vi "CH_LM App DAQ SendCommand.vi"(4 "error in (no error)":errorcluster, 5 "DAQ Command":T1={"Wait at Rendesvouz"=FALSE, "Command"="", "Sample Collection"=enum."Continuous", "Sample Size"=100, "Collection Mode"=enum."Streaming", "T / ms"=1.0, "NofBins"=7, "Point(s)"=1, "Log Data File"=path "", "Log data to File"=FALSE, "Pause"=FALSE, "Meter Index"=0, "Data format"=0, "Delivery Mode"=enum."Last", "Start/Stop Button"=refnum, "Point(s) Array"=[]} {"Point(s) Array" min=1 max=20000; "Point(s)" min=1 max=20000; "Sample Size" min=1}, 6 "rendezvous":T3, 7 "i ref":refnum<vi>) -> (0 "error out":errorcluster, 2 "timed out":bool, 3 "i ref":refnum<vi>)   [LabVIEW 2012, in "CH_LM App.lvlib"]
doc: "This VI can be used to send a command to the DAQ thread."
uses:
  CH_LM App.lvlib
  CH_LM App DAQ Command.ctl
  CH_LM/CH_LM Measurement Delivery Mode.ctl
  CH_LM.lvlib
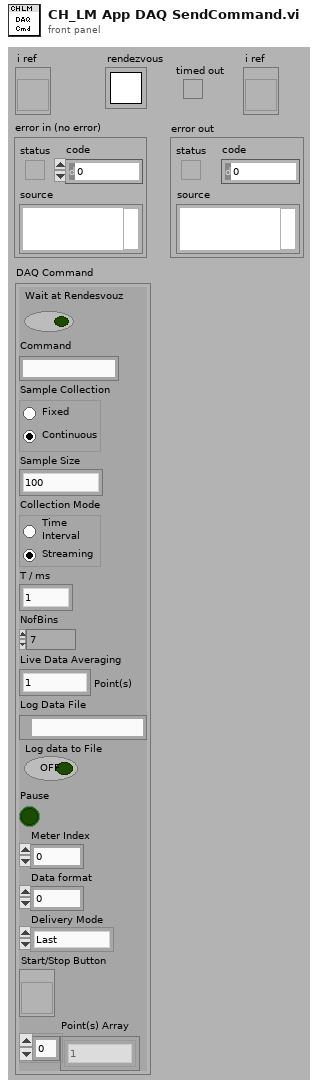
[diagram p1: front panel]
types:
  T1 = typedef "CH_LM App.lvlib/CH_LM App DAQ Command.ctl" = cluster{"Wait at Rendesvouz":bool, "Command":string, "Sample Collection":enum32{"Fixed", "Continuous"}, "Sample Size":i32, "Collection Mode":enum32{"Time\nInterval", "Streaming"}, "T / ms":dbl, "NofBins":i32, "Point(s)":u32, "Log Data File":path, "Log data to File":bool, "Pause":bool, "Meter Index":i32, "Data format":u16, "Delivery Mode":T2, "Start/Stop Button":refnum<vi>, "Point(s) Array":u32[]}
  T2 = typedef "CH_LM.lvlib/CH_LM Measurement Delivery Mode.ctl" = enum16{"Last", "Stream"}
  T3 = typedef "Rendezvous RefNum" = refnum<k1>
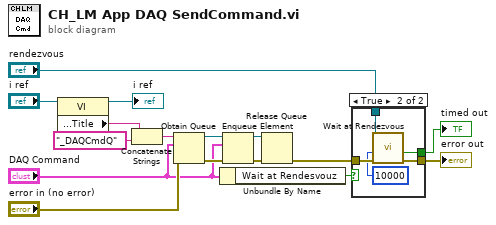
[diagram p0: block diagram]
diagram:
  n1 = property on="Property Node" class="VI"(reference="i ref") -> ("Front Panel Window:Title"=w12:string)  [unwired: 1 in, 2 out]
  n2 = Concatenate Strings(w12, "_DAQCmdQ" ("string")) -> (w6:string)
  n3 = Obtain Queue(name (unnamed)=w6, element data type="DAQ Command", error in (no error)="error in (no error)") -> (queue out=w8:refnum<queue>, error out=w9:errorcluster)  [unwired: 2 in, 1 out]
  n4 = Unbundle By Name("DAQ Command") -> ("Wait at Rendesvouz"=w2:bool)
  n5 = Enqueue Element(queue=w8, element="DAQ Command", error in (no error)=w9) -> (queue out=w10:refnum<queue>, error out=w11:errorcluster)  [unwired: 2 out]
  n6 = Release Queue(queue=w10, error in (no error)=w11) -> (error out=w13:errorcluster)  [unwired: 3 out]
  n7 = case shown="True" w2 {
    tunnel: "rendezvous" -> [_ w21]
    tunnel: [w16 w20] -> w14
    tunnel: w13 -> [w16 w19]
    tunnel: [_ w17] -> w5
    frame False {
    }
    frame True {
      n8 = call <vilib>:"Wait at Rendezvous.vi"("error in (no error)"=w19, "ms timeout (-1)"=10000, "rendezvous"=w21) -> ("error out"=w20:errorcluster, "timed out"=w17:bool)  [unwired: 3 out]
    }
  }
  "error out" <- w14
  "timed out" <- w5
  "i ref" <- "i ref"
